vi "Get Message TypeUrl.vi"(8 "error in (no error)":errorcluster, 11 "Message ref in":u64) -> (0 "error out":errorcluster, 1 "Message Name":string, 3 "Message ref out":u64)   [LabVIEW 2019, in "gRPC Scripting Tools.lvlib"]
uses:
  gRPC Scripting Tools.lvlib
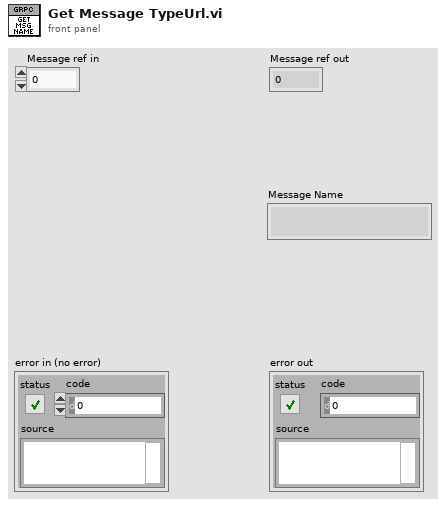
[diagram p1: front panel]
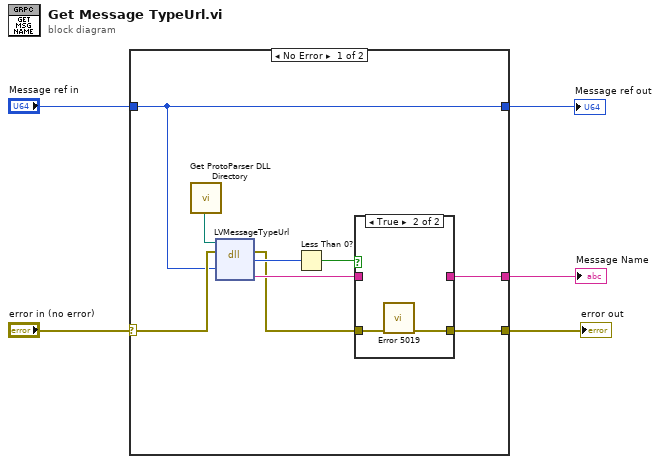
[diagram p0: block diagram]
diagram:
  n1 = case shown="No Error" "error in (no error)" {
    selector: "error in (no error)" -> [w13 w20]
    tunnel: "Message ref in" -> [w12 w19]
    tunnel: [w12 w19] -> w3
    tunnel: [w6 w20] -> w2
    tunnel: [w10 _] -> w1
    frame No Error {
      n2 = call "Get ProtoParser DLL Directory.vi"() -> ("Proto Parser Directory"=w14:path)
      n3 = dll-call lib="C:/Users/XEnderMD/Desktop/LV gRPC/labview source/gRPC Scripting Tools/Proto Parser API/dll/labview_grpc_generator.dll" fn="LVMessageTypeUrl"(path in=w14, error in=w13, "message"=w12) -> (error out=w7:errorcluster, "return type"=w9:i32, "name"=w11:string)  [unwired: 3 in, 1 out]
      n4 = Less Than 0?(x=w9) -> (x < 0?=w8:bool)
      n5 = case shown="True" w8 {
        tunnel: w11 -> [w15 _]
        tunnel: [w15 _] -> w10
        tunnel: w7 -> [w16 w18]
        tunnel: [w16 w17] -> w6
        frame False {
        }
        frame True {
          n6 = call "Error 5019.vi"("error in (no error)"=w18) -> ("error out"=w17:errorcluster)  [unwired: 10 in]
        }
      }
    }
    frame Error {
    }
  }
  "Message Name" <- w1
  "Message ref out" <- w3
  "error out" <- w2
